vi "SelectMenu5.vi"(0 "XRef":T21, 1 "Tag":T16, 2 "Point":T19, 3 "Menu Type":T18, 4 "State In":T1={"Worker Library Path"=path "", "Block Label"="", "Types"=[], "Selections"=[], "Icon"={"image type"=0, "image depth"=0, "image"=[], "mask"=[], "colors"=[], "Rectangle"={"left"=0, "top"=0, "right"=0, "bottom"=0}}, "Errors"={"Terminals"=[], "Generate"={"status"=FALSE, "code"=0, "source"=""}, "General"={"status"=FALSE, "code"=0, "source"=""}}, "Calculated Sizes"={"Block Width"=0, "Block Height"=0, "Half Width"=0, "Icon Top"=0, "Icon Bottom"=0, "Label Width"=0, "Half Label"=0, "Label Top"=0, "Text Width"=0, "Half Text"=0, "Text Height"=0, "Label Height"=0, "Expanded Width"=0, "Label Bottom"=0, "Expanded Top"=0, "Expanded Bottom"=0, "Expanded Height"=0, "Min Height"=0, "Max Height"=0}, "Special Terminal Indices"={"Action"=-1, "Init"=-1, "Tag"=-1, "State in"=-1, "State out"=-1, "Error"=-1, "Control"=-1, "Config"=-1}, "Terminals"=[], "Temp VI Name"="", "Description"="", "Smol Mode"=FALSE}) -> (14 "Reply":T15, 15 "Handled?":T17, 16 "Multi Object Popup Options":T14, 17 "Fatal Error Out":T13, 18 "State Out":T1={"Worker Library Path"=path "", "Block Label"="", "Types"=[], "Selections"=[], "Icon"={"image type"=0, "image depth"=0, "image"=[], "mask"=[], "colors"=[], "Rectangle"={"left"=0, "top"=0, "right"=0, "bottom"=0}}, "Errors"={"Terminals"=[], "Generate"={"status"=FALSE, "code"=0, "source"=""}, "General"={"status"=FALSE, "code"=0, "source"=""}}, "Calculated Sizes"={"Block Width"=0, "Block Height"=0, "Half Width"=0, "Icon Top"=0, "Icon Bottom"=0, "Label Width"=0, "Half Label"=0, "Label Top"=0, "Text Width"=0, "Half Text"=0, "Text Height"=0, "Label Height"=0, "Expanded Width"=0, "Label Bottom"=0, "Expanded Top"=0, "Expanded Bottom"=0, "Expanded Height"=0, "Min Height"=0, "Max Height"=0}, "Special Terminal Indices"={"Action"=-1, "Init"=-1, "Tag"=-1, "State in"=-1, "State out"=-1, "Error"=-1, "Control"=-1, "Config"=-1}, "Terminals"=[], "Temp VI Name"="", "Description"="", "Smol Mode"=FALSE})   [LabVIEW 2022 SP3, in "Flex Block.xnode"]
uses:
  Flex Block.xnode
  FlexBlocks Support/FlexBlocks Support.lvlib
  <vilib>/Utility/miscctls.llb/LVPositionTypeDef.ctl
  FlexBlocks Support/Write Terminals.ctl
  FlexBlocks Support/Lossy Terminals.ctl
  FlexBlocks Support/Lossless Terminals.ctl
  FlexBlocks Support/Event Terminals.ctl
  <vilib>/XNodeSupport/XNodeXNodeRef.ctl
  <vilib>/XNodeSupport/NI_XNodeSupport.lvlib
  <vilib>/XNodeSupport/XNodeString.ctl
  <vilib>/XNodeSupport/XNodeInt.ctl
  <vilib>/XNodeSupport/XNodePoint.ctl
  <vilib>/XNodeSupport/XNodeMenuType.ctl
  <vilib>/XNodeSupport/XNodeStringArray.ctl
  <vilib>/XNodeSupport/XNodeBool.ctl
  <vilib>/XNodeSupport/XNodeMultiObjectPopupOptions.ctl
  <vilib>/XNodeSupport/XNodeErrorCluster.ctl
  State.ctl
  FlexBlocks Support/Terminal Direction.ctl
  FlexBlocks Support/Value Mode.ctl
  FlexBlocks Support/Special Terminal.ctl
  FlexBlocks Support/Type Descriptor.ctl
  <vilib>/picture/picture.llb/imagedata.ctl
  FlexBlocks Support/XNode Errors.ctl
  FlexBlocks Support/Calculated Sizes.ctl
  FlexBlocks Support/Special Terminal Indices.ctl
  FlexBlocks Support/Terminal State.ctl
  FlexBlocks Support/Terminal Status.ctl
  FlexBlocks Support/Terminal Draw Style.ctl
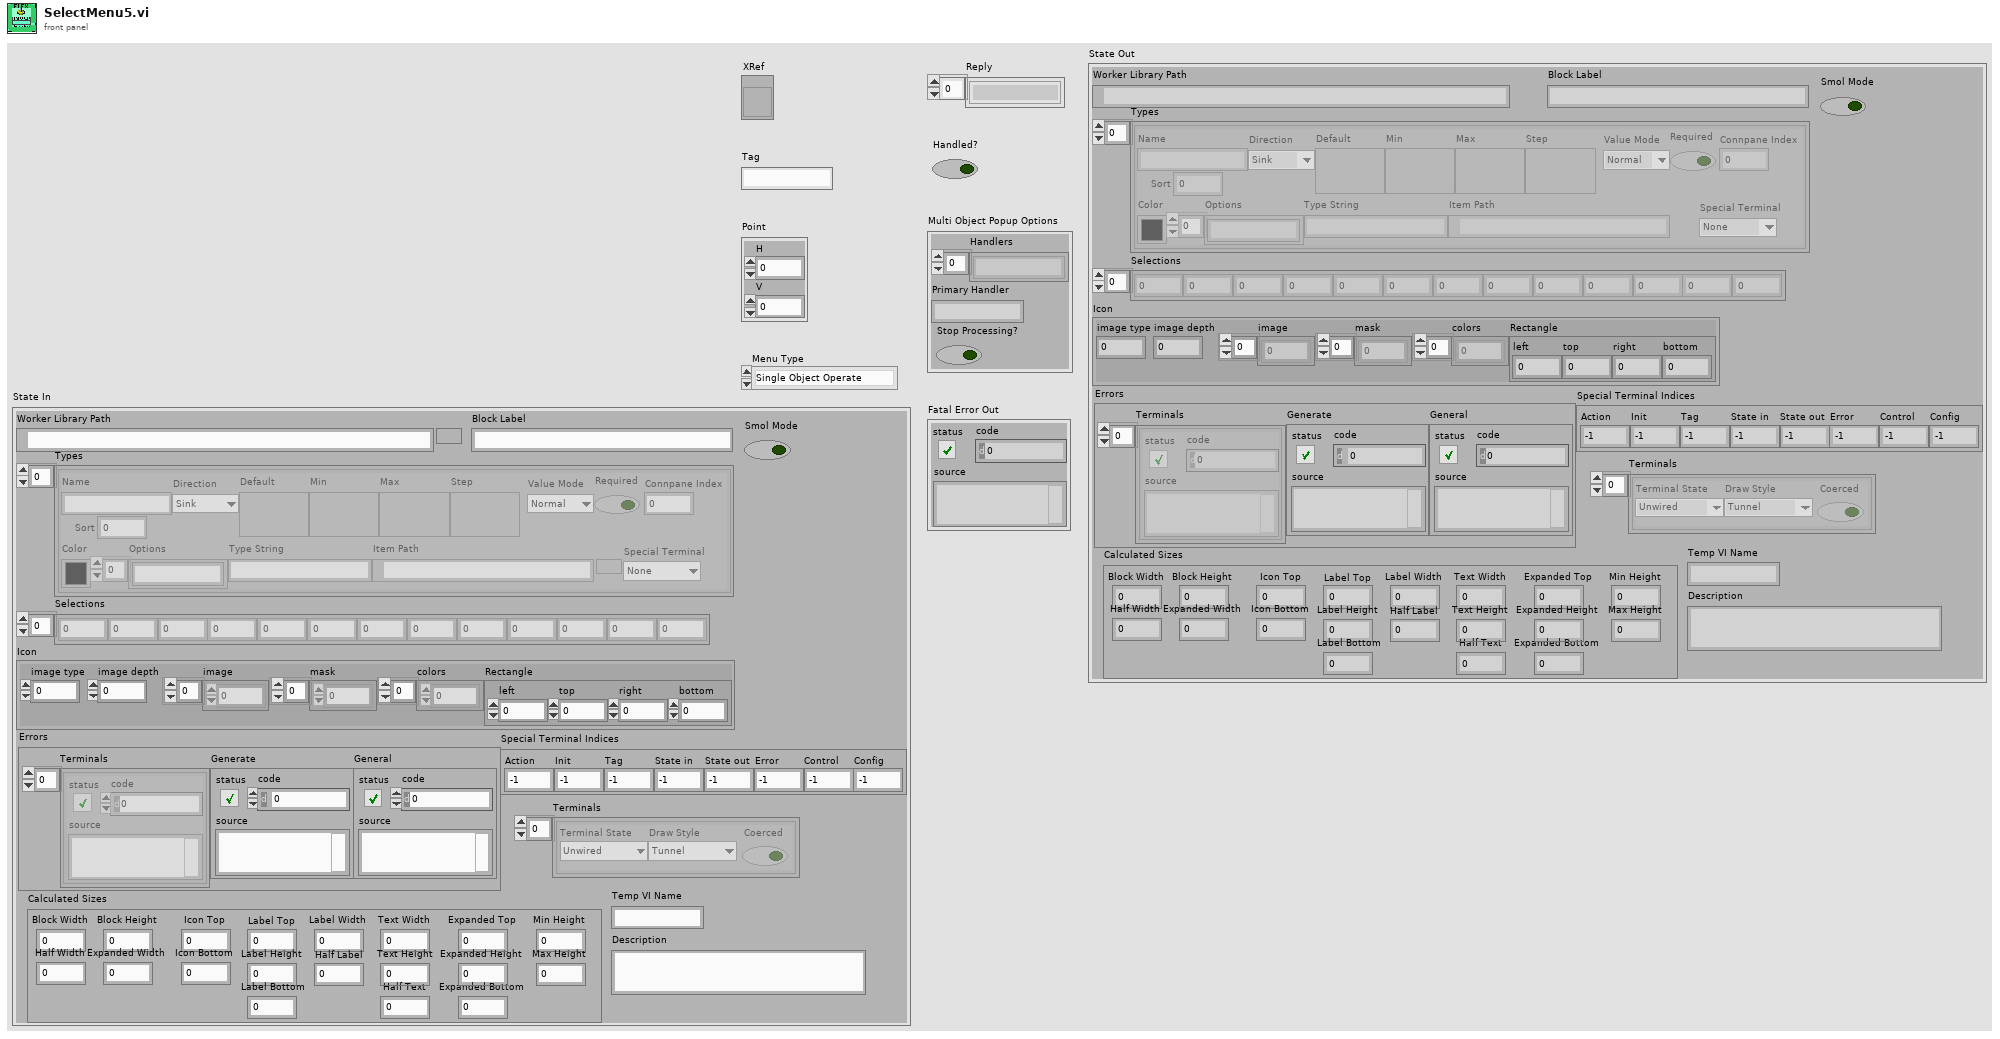
[diagram p1: front panel]
types:
  T1 = typedef "Flex Block.xnode/State.ctl" = cluster{"Worker Library Path":path, "Block Label":string, "Types":T2[], "Selections":i32[], "Icon":T6, "Errors":T7, "Calculated Sizes":T8, "Special Terminal Indices":T9, "Terminals":T10[], "Temp VI Name":string, "Description":string, "Smol Mode":bool}
  T2 = typedef "FlexBlocks Support.lvlib/Type Descriptor.ctl" = cluster{"Name":string, "Direction":T3, "Default":variant, "Min":variant, "Max":variant, "Step":variant, "Value Mode":T4, "Color":u32, "Options":string[], "Type String":string, "Item Path":path, "Required":bool, "Connpane Index":i32, "Special Terminal":T5, "Sort":i32}
  T3 = typedef "FlexBlocks Support.lvlib/Terminal Direction.ctl" = enum16{"Sink", "Source"}
  T4 = typedef "FlexBlocks Support.lvlib/Value Mode.ctl" = enum16{"Normal", "Range", "Select"}
  T5 = typedef "FlexBlocks Support.lvlib/Special Terminal.ctl" = enum16{"None", "Action", "Init", "Tag", "State in", "State out", "Error", "Control", "Config"}
  T6 = typedef "imagedata.ctl" = cluster{"image type":i32, "image depth":i32, "image":u8[], "mask":u8[], "colors":u32[], "Rectangle":cluster{"left":i16, "top":i16, "right":i16, "bottom":i16}}
  T7 = typedef "FlexBlocks Support.lvlib/XNode Errors.ctl" = cluster{"Terminals":errorcluster[], "Generate":errorcluster, "General":errorcluster}
  T8 = typedef "FlexBlocks Support.lvlib/Calculated Sizes.ctl" = cluster{"Block Width":i32, "Block Height":i32, "Half Width":i32, "Icon Top":i32, "Icon Bottom":i32, "Label Width":i32, "Half Label":i32, "Label Top":i32, "Text Width":i32, "Half Text":i32, "Text Height":i32, "Label Height":i32, "Expanded Width":i32, "Label Bottom":i32, "Expanded Top":i32, "Expanded Bottom":i32, "Expanded Height":i32, "Min Height":i32, "Max Height":i32}
  T9 = typedef "FlexBlocks Support.lvlib/Special Terminal Indices.ctl" = cluster{"Action":i32, "Init":i32, "Tag":i32, "State in":i32, "State out":i32, "Error":i32, "Control":i32, "Config":i32}
  T10 = typedef "FlexBlocks Support.lvlib/Terminal Status.ctl" = cluster{"Terminal State":T11, "Draw Style":T12, "Coerced":bool}
  T11 = typedef "FlexBlocks Support.lvlib/Terminal State.ctl" = enum16{"Unwired", "BadType", "BadRef", "Channel", "Value", "Control Ref"}
  T12 = typedef "FlexBlocks Support.lvlib/Terminal Draw Style.ctl" = enum16{"Tunnel", "BadType", "BadRef", "Channel", "Value", "Control Ref"}
  T13 = typedef "NI_XNodeSupport.lvlib/XNodeErrorCluster.ctl" = errorcluster
  T14 = typedef "NI_XNodeSupport.lvlib/XNodeMultiObjectPopupOptions.ctl" = cluster{"Handlers":T15, "Primary Handler":T16, "Stop Processing?":T17}
  T15 = typedef "NI_XNodeSupport.lvlib/XNodeStringArray.ctl" = T16[]
  T16 = typedef "NI_XNodeSupport.lvlib/XNodeString.ctl" = string
  T17 = typedef "NI_XNodeSupport.lvlib/XNodeBool.ctl" = bool
  T18 = typedef "NI_XNodeSupport.lvlib/XNodeMenuType.ctl" = enum32{"Single Object Operate", "Single Object Popup", "Multi Object Popup Master", "Multi Object Popup Other"}
  T19 = typedef "NI_XNodeSupport.lvlib/XNodePoint.ctl" = cluster{"H":T20, "V":T20}
  T20 = typedef "NI_XNodeSupport.lvlib/XNodeInt.ctl" = i32
  T21 = typedef "NI_XNodeSupport.lvlib/XNodeXNodeRef.ctl" = refnum<vi>
  T22 = typedef "FlexBlocks Support.lvlib/Menu Tag.ctl" = enum16{"Unknown", "Create Channel Writer", "Create Lossy Reader", "Create Lossless Reader", "Create Event Reader", "Smol Mode", "Open Block VI", "Open Block Library", "Create Null Terminal"}
  T23 = typedef "FlexBlocks Support.lvlib/Write Terminals.ctl" = enum16{"Timeout mS", "NC 1", "Element", "Close", "Pause", "Timed Out?", "NC 6", "FlexChannel", "Closed?"}
  T24 = typedef "LVPositionTypeDef.ctl" = cluster{"Left":i32, "Top":i32}
  T25 = typedef "FlexBlocks Support.lvlib/Lossy Terminals.ctl" = enum16{"Wait for Next?", "Updated", "FlexChannel", "Wait Timeout mS", "New Value?", "Timed Out?", "NC 6", "Value", "Closed?"}
  T26 = typedef "FlexBlocks Support.lvlib/Lossless Terminals.ctl" = enum16{"Depth", "Timeout mS", "FlexChannel", "Release", "Restart", "Paused?", "Timed Out?", "Element", "Close", "Closed?"}
  T27 = typedef "FlexBlocks Support.lvlib/Event Terminals.ctl" = enum16{"NC 0", "NC 1", "FlexChannel", "NC 3", "NC 4", "NC 5", "NC 6", "Event Reg"}
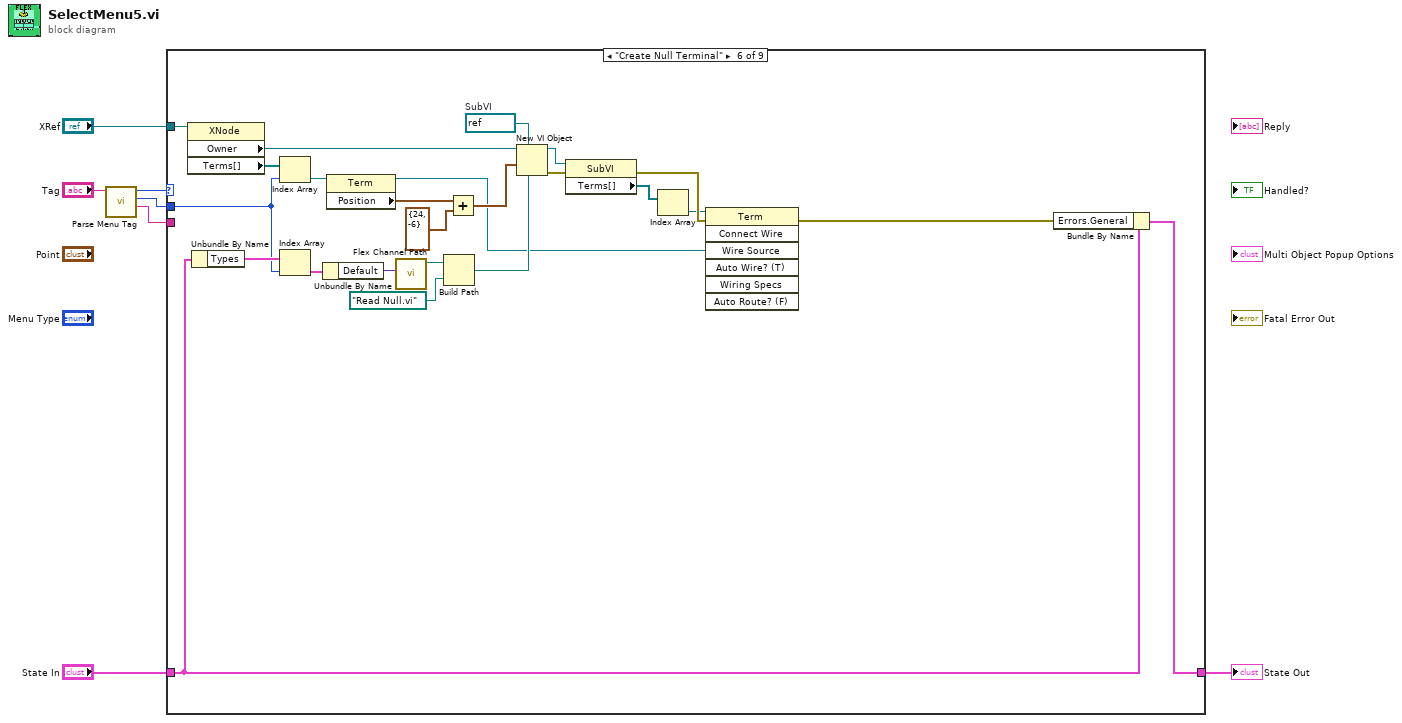
[diagram p0: block diagram]
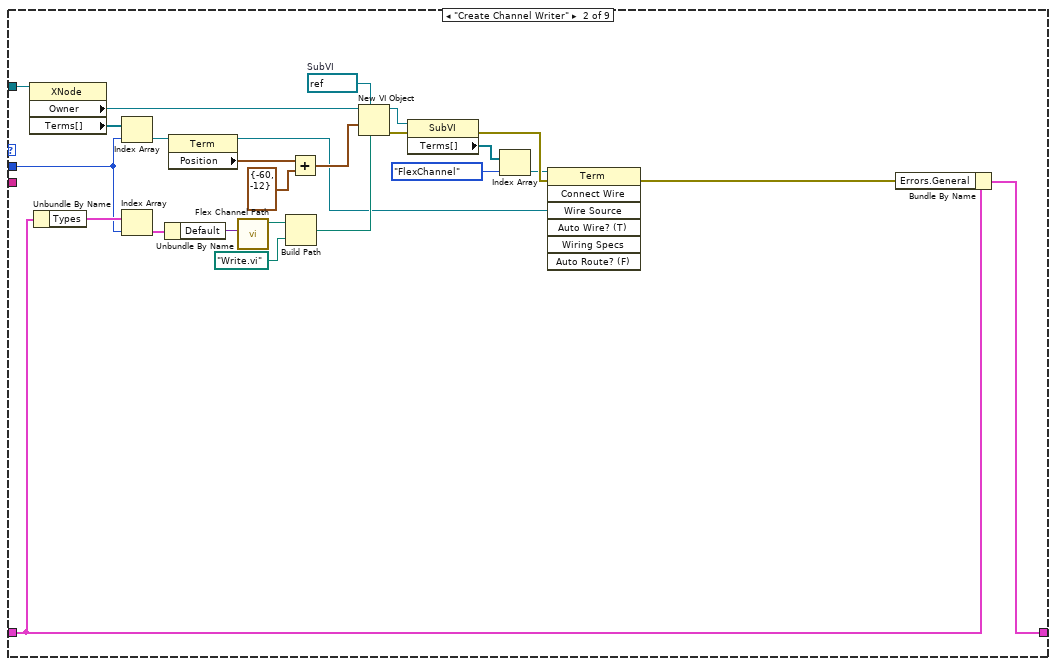
[diagram p3: hidden frame]
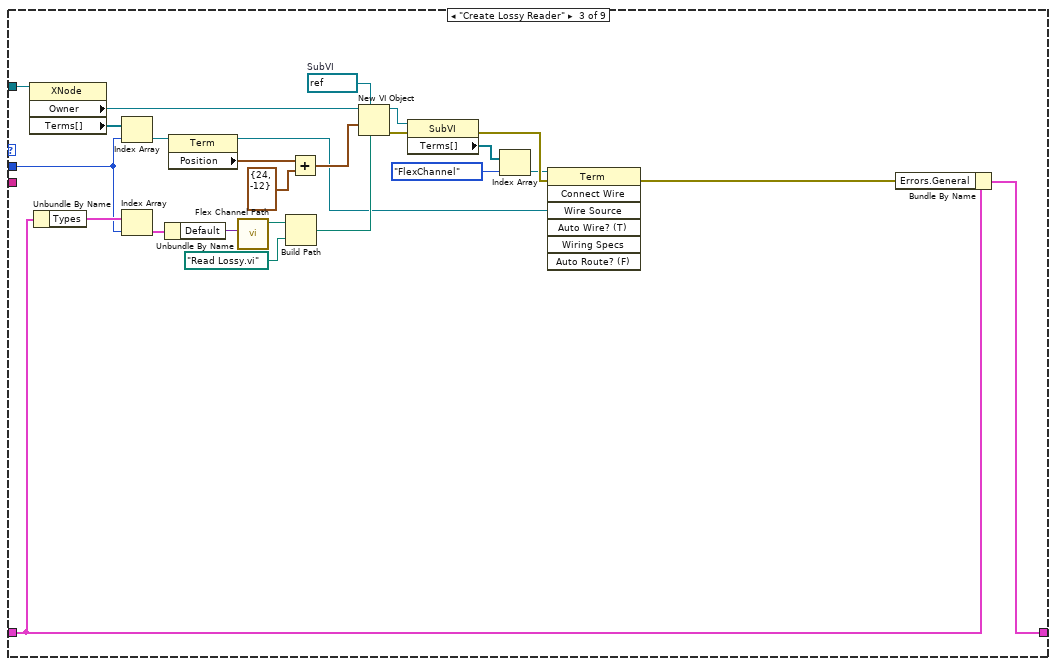
[diagram p4: hidden frame]
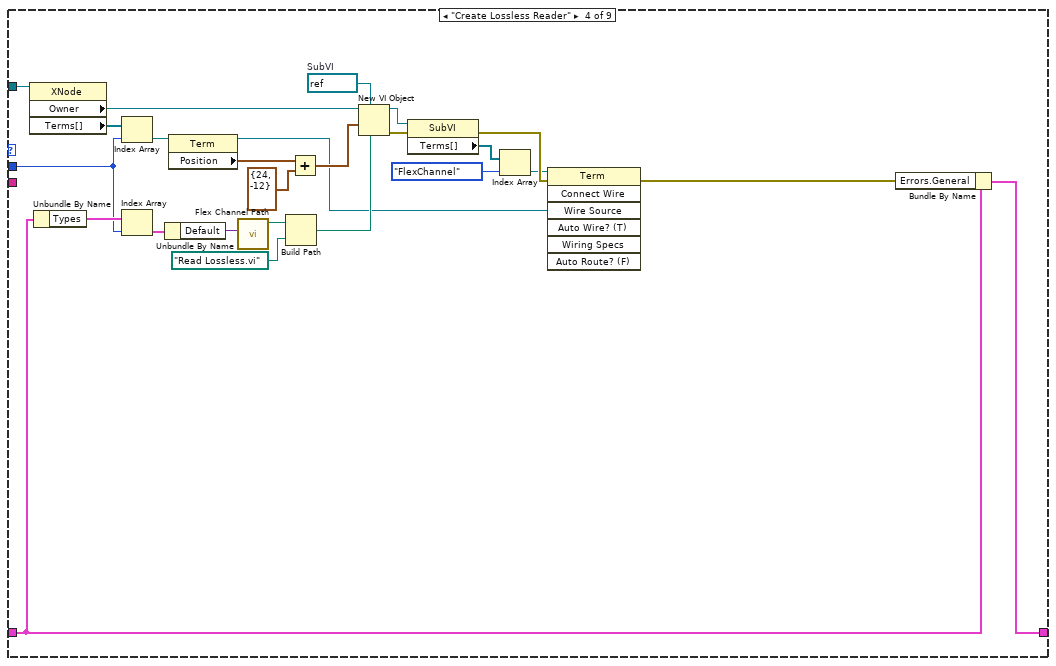
[diagram p5: hidden frame]
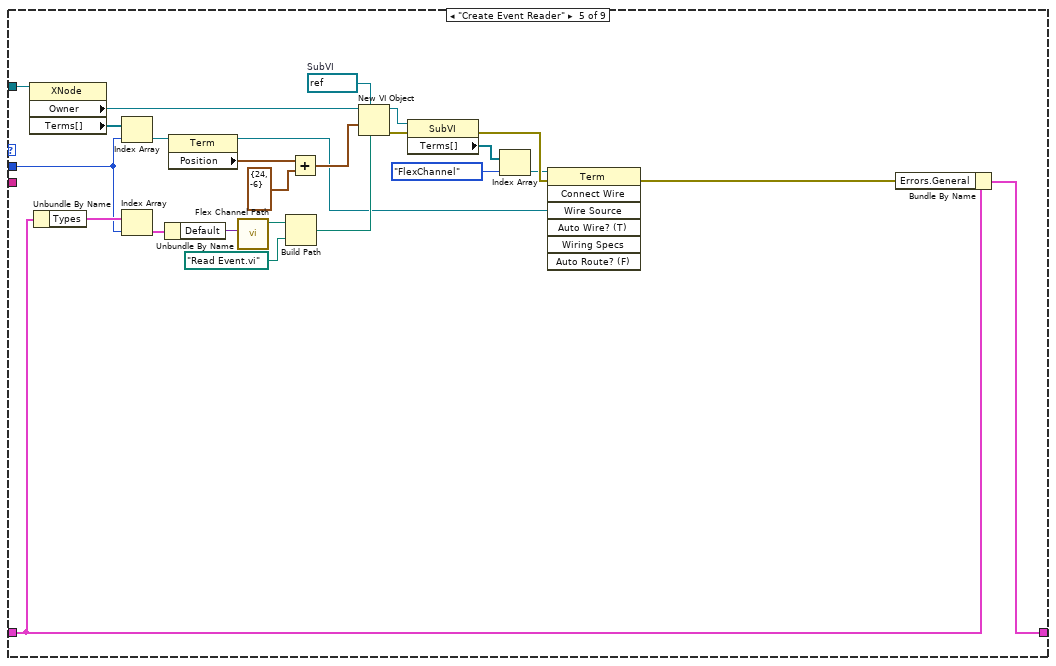
[diagram p6: hidden frame]
diagram:
  n1 = call "Parse Menu Tag.vi"("Tag"="Tag") -> ("String"=w2:string, "Int"=w3:i32, "Menu Tag"=w4:T22)  [unwired: 8 in]
  n2 = case shown="\"Create Null Terminal\"" w4 {
    tunnel: "State In" -> [w8 w16 w41 w66 w91 w115 w133 w134 w135]
    tunnel: [w8 w17 w42 w67 w92 w116 w133 w134 w135] -> w6
    tunnel: w3 -> [_ w29 w54 w79 w104 w128 _ _ _]
    tunnel: w2 -> [_ _ _ _ _ _ _ _ _]
    tunnel: "XRef" -> [_ w32 w57 w82 w107 w131 _ _ _]
    frame "Unknown" {
      # "Not one of our tags, should this be an error?"
    }
    frame "Create Channel Writer" {
      w22 = refnum<vi> refnum  # SubVI
      n3 = property class="XNode"(reference=w32) -> ("Owner"=w23:refnum<vi>, "Terms[]"=w30:refnum<vi>[])  [unwired: 1 in, 2 out]
      n4 = Unbundle By Name(w16) -> ("Types"=w31:T2[])
      n5 = Index Array(array=w30, index=w29) -> (element=w24:refnum<vi>)
      n6 = Index Array(array=w31, index=w29) -> (element=w28:T2)
      n7 = Unbundle By Name(w28) -> ("Default"=w27:variant)
      n8 = property class="Term"(reference=w24) -> (reference out=w10:refnum<vi>, "Position"=w20:T24)  [unwired: 1 in, 1 out]
      n9 = call "Flex Channel Path.vi"("Variant"=w27) -> ("Channel Folder Path"=w26:path)  [unwired: 9 in, 1 out]
      n10 = Build Path(base path=w26, name or relative path=path "Write.vi") -> (appended path=w21:path)
      n11 = Add(x=w20, y=T24 {"Left"=-60, "Top"=-12} ("Position")) -> (x+y=w18:T24)
      n12 = New VI Object(vi object class=w22, owner refnum=w23, position/next to=w18, 6:w21) -> (object refnum=w14:refnum<vi>, 0:w15:errorcluster)  [unwired: 4 in]
      n13 = property class="SubVI"(reference=w14, error in=w15) -> (error out=w33:errorcluster, "Terms[]"=w13:refnum<vi>[])  [unwired: 1 out]
      n14 = Index Array(array=w13, index=Write_Terminals."FlexChannel" ("Write Terminals")) -> (element=w11:refnum<vi>)
      n15 = invoke class="Term" method="Connect Wire"(reference=w11, error in=w33, "Wire Source"=w10) -> (error out=w9:errorcluster)  [unwired: 4 in, 6 out]
      n16 = Bundle By Name(cluster=w16, "Errors.General"=w9) -> (w17:T1)
    }
    frame "Create Lossy Reader" {
      w47 = refnum<vi> refnum  # SubVI
      n17 = property class="XNode"(reference=w57) -> ("Owner"=w48:refnum<vi>, "Terms[]"=w55:refnum<vi>[])  [unwired: 1 in, 2 out]
      n18 = Unbundle By Name(w41) -> ("Types"=w56:T2[])
      n19 = Index Array(array=w55, index=w54) -> (element=w49:refnum<vi>)
      n20 = Index Array(array=w56, index=w54) -> (element=w53:T2)
      n21 = Unbundle By Name(w53) -> ("Default"=w52:variant)
      n22 = property class="Term"(reference=w49) -> (reference out=w35:refnum<vi>, "Position"=w45:T24)  [unwired: 1 in, 1 out]
      n23 = call "Flex Channel Path.vi"("Variant"=w52) -> ("Channel Folder Path"=w51:path)  [unwired: 9 in, 1 out]
      n24 = Build Path(base path=w51, name or relative path=path "Read Lossy.vi") -> (appended path=w46:path)
      n25 = Add(x=w45, y=T24 {"Left"=24, "Top"=-12} ("Position")) -> (x+y=w43:T24)
      n26 = New VI Object(vi object class=w47, owner refnum=w48, position/next to=w43, 6:w46) -> (object refnum=w39:refnum<vi>, 0:w40:errorcluster)  [unwired: 4 in]
      n27 = property class="SubVI"(reference=w39, error in=w40) -> (error out=w58:errorcluster, "Terms[]"=w38:refnum<vi>[])  [unwired: 1 out]
      n28 = Index Array(array=w38, index=Lossy_Terminals."FlexChannel" ("Lossy Terminals")) -> (element=w36:refnum<vi>)
      n29 = invoke class="Term" method="Connect Wire"(reference=w36, error in=w58, "Wire Source"=w35) -> (error out=w34:errorcluster)  [unwired: 4 in, 6 out]
      n30 = Bundle By Name(cluster=w41, "Errors.General"=w34) -> (w42:T1)
    }
    frame "Create Lossless Reader" {
      w72 = refnum<vi> refnum  # SubVI
      n31 = property class="XNode"(reference=w82) -> ("Owner"=w73:refnum<vi>, "Terms[]"=w80:refnum<vi>[])  [unwired: 1 in, 2 out]
      n32 = Unbundle By Name(w66) -> ("Types"=w81:T2[])
      n33 = Index Array(array=w80, index=w79) -> (element=w74:refnum<vi>)
      n34 = Index Array(array=w81, index=w79) -> (element=w78:T2)
      n35 = Unbundle By Name(w78) -> ("Default"=w77:variant)
      n36 = property class="Term"(reference=w74) -> (reference out=w60:refnum<vi>, "Position"=w70:T24)  [unwired: 1 in, 1 out]
      n37 = call "Flex Channel Path.vi"("Variant"=w77) -> ("Channel Folder Path"=w76:path)  [unwired: 9 in, 1 out]
      n38 = Build Path(base path=w76, name or relative path=path "Read Lossless.vi") -> (appended path=w71:path)
      n39 = Add(x=w70, y=T24 {"Left"=24, "Top"=-12} ("Position")) -> (x+y=w68:T24)
      n40 = New VI Object(vi object class=w72, owner refnum=w73, position/next to=w68, 6:w71) -> (object refnum=w64:refnum<vi>, 0:w65:errorcluster)  [unwired: 4 in]
      n41 = property class="SubVI"(reference=w64, error in=w65) -> (error out=w83:errorcluster, "Terms[]"=w63:refnum<vi>[])  [unwired: 1 out]
      n42 = Index Array(array=w63, index=Lossless_Terminals."FlexChannel" ("Lossless Terminals")) -> (element=w61:refnum<vi>)
      n43 = invoke class="Term" method="Connect Wire"(reference=w61, error in=w83, "Wire Source"=w60) -> (error out=w59:errorcluster)  [unwired: 4 in, 6 out]
      n44 = Bundle By Name(cluster=w66, "Errors.General"=w59) -> (w67:T1)
    }
    frame "Create Event Reader" {
      w97 = refnum<vi> refnum  # SubVI
      n45 = property class="XNode"(reference=w107) -> ("Owner"=w98:refnum<vi>, "Terms[]"=w105:refnum<vi>[])  [unwired: 1 in, 2 out]
      n46 = Unbundle By Name(w91) -> ("Types"=w106:T2[])
      n47 = Index Array(array=w105, index=w104) -> (element=w99:refnum<vi>)
      n48 = Index Array(array=w106, index=w104) -> (element=w103:T2)
      n49 = Unbundle By Name(w103) -> ("Default"=w102:variant)
      n50 = property class="Term"(reference=w99) -> (reference out=w85:refnum<vi>, "Position"=w95:T24)  [unwired: 1 in, 1 out]
      n51 = call "Flex Channel Path.vi"("Variant"=w102) -> ("Channel Folder Path"=w101:path)  [unwired: 9 in, 1 out]
      n52 = Build Path(base path=w101, name or relative path=path "Read Event.vi") -> (appended path=w96:path)
      n53 = Add(x=w95, y=T24 {"Left"=24, "Top"=-6} ("Position")) -> (x+y=w93:T24)
      n54 = New VI Object(vi object class=w97, owner refnum=w98, position/next to=w93, 6:w96) -> (object refnum=w89:refnum<vi>, 0:w90:errorcluster)  [unwired: 4 in]
      n55 = property class="SubVI"(reference=w89, error in=w90) -> (error out=w108:errorcluster, "Terms[]"=w88:refnum<vi>[])  [unwired: 1 out]
      n56 = Index Array(array=w88, index=Event_Terminals."FlexChannel" ("Event Terminals")) -> (element=w86:refnum<vi>)
      n57 = invoke class="Term" method="Connect Wire"(reference=w86, error in=w108, "Wire Source"=w85) -> (error out=w84:errorcluster)  [unwired: 4 in, 6 out]
      n58 = Bundle By Name(cluster=w91, "Errors.General"=w84) -> (w92:T1)
    }
    frame "Create Null Terminal" {
      w121 = refnum<vi> refnum  # SubVI
      n59 = property class="XNode"(reference=w131) -> ("Owner"=w122:refnum<vi>, "Terms[]"=w129:refnum<vi>[])  [unwired: 1 in, 2 out]
      n60 = Unbundle By Name(w115) -> ("Types"=w130:T2[])
      n61 = Index Array(array=w129, index=w128) -> (element=w123:refnum<vi>)
      n62 = Index Array(array=w130, index=w128) -> (element=w127:T2)
      n63 = Unbundle By Name(w127) -> ("Default"=w126:variant)
      n64 = property class="Term"(reference=w123) -> (reference out=w110:refnum<vi>, "Position"=w119:T24)  [unwired: 1 in, 1 out]
      n65 = call "Flex Channel Path.vi"("Variant"=w126) -> ("Channel Folder Path"=w125:path)  [unwired: 9 in, 1 out]
      n66 = Build Path(base path=w125, name or relative path=path "Read Null.vi") -> (appended path=w120:path)
      n67 = Add(x=w119, y=T24 {"Left"=24, "Top"=-6} ("Position")) -> (x+y=w117:T24)
      n68 = New VI Object(vi object class=w121, owner refnum=w122, position/next to=w117, 6:w120) -> (object refnum=w113:refnum<vi>, 0:w114:errorcluster)  [unwired: 4 in]
      n69 = property class="SubVI"(reference=w113, error in=w114) -> (error out=w132:errorcluster, "Terms[]"=w112:refnum<vi>[])  [unwired: 1 out]
      n70 = Index Array(array=w112) -> (element=w111:refnum<vi>)  [unwired: 1 in]
      n71 = invoke class="Term" method="Connect Wire"(reference=w111, error in=w132, "Wire Source"=w110) -> (error out=w109:errorcluster)  [unwired: 4 in, 6 out]
      n72 = Bundle By Name(cluster=w115, "Errors.General"=w109) -> (w116:T1)
    }
    frame "Smol Mode" {
    }
    frame "Open Block VI" {
    }
    frame "Open Block Library" {
    }
  }
  "State Out" <- w6
